vi "TestArena.vi"() -> ()   [LabVIEW 2013]
panel:
  out "Direction Command":bool
  in  "Motor PWM Request":dbl
  in  "Direction Request":bool
  out "Motor PWM Command":dbl
  out "Direction Enabled":bool caption="Time has Elapsed"
  in  "stop":bool
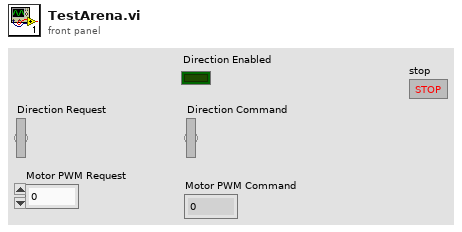
[diagram p1: front panel]
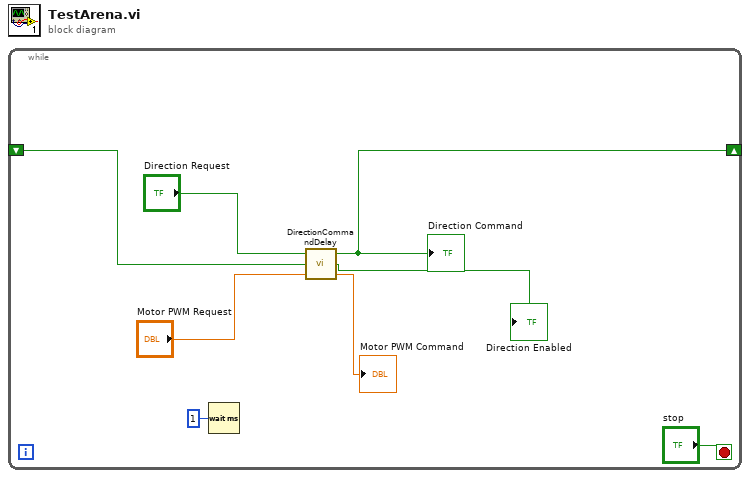
[diagram p0: block diagram]
diagram:
  n1 = while {
    shift-right: [w2] -> _
    shift-left: _ -> [w4]
    stop <- "stop" stop-if-true
    n2 = Wait (ms)(milliseconds to wait=u32 1) -> ()  [unwired: 1 out]
    n3 = call "DirectionCommandDelay.vi"("Motor PWM Request"="Motor PWM Request", "Current Direction"=w4, "Direction Request"="Direction Request") -> ("Motor PWM Command"=→"Motor PWM Command":dbl, "Direction Enabled"=→"Direction Enabled":bool, "Direction Command"=w2:bool)
    "Direction Command" <- w2
  }
